vi "Calculate limits based on percent tolerance.vi"(4 "Tolerance %":dbl, 5 "Value":dbl) -> (1 "Low":dbl, 2 "High":dbl)   [LabVIEW 2020]
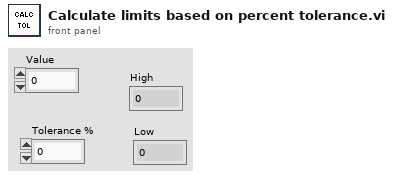
[diagram p1: front panel]
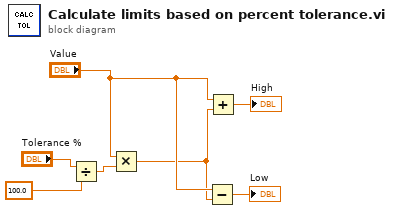
[diagram p0: block diagram]
diagram:
  n1 = Divide(x="Tolerance %", y=100.0) -> (x/y=w5:dbl)
  n2 = Multiply(x="Value", y=w5) -> (x*y=w3:dbl)
  n3 = Subtract(x="Value", y=w3) -> (x-y=→"Low":dbl)
  n4 = Add(x="Value", y=w3) -> (x+y=→"High":dbl)
